vi "tcpserver.vi"   [LabVIEW 2016]
uses:
  executables/arguments.ctl
types:
  T1 = typedef "arguments.ctl" = cluster{"working directory":string, "flags":string[], "values":string[]}
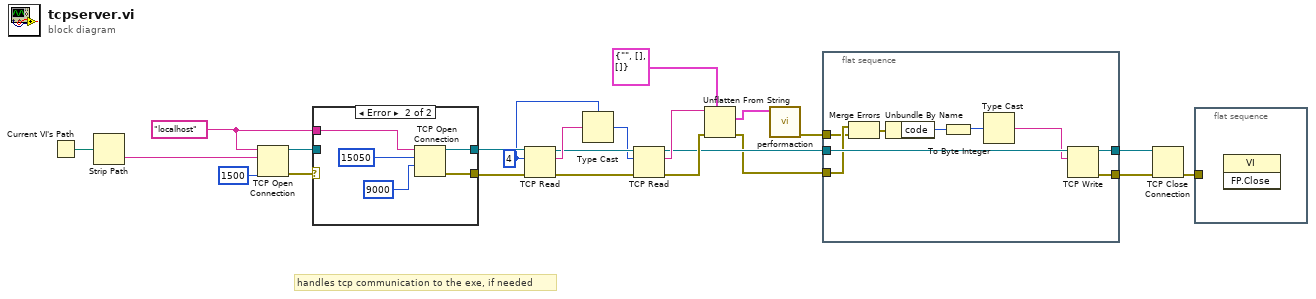
[diagram p0: block diagram]
diagram:
  w17 = 4 ("bytes to read")
  w20 = "localhost" ("address")
  # "handles tcp communication to the exe, if needed"
  n1 = Current VI's Path() -> (path=w3:path)
  n2 = Strip Path(path=w3) -> (name=w2:string)  [unwired: 1 out]
  n3 = TCP Open Connection(address=w20, remote port or service name=w2, timeout ms (60000)=1500) -> (connection ID=w21:refnum<k5>, error out=w22:errorcluster)  [unwired: 2 in]
  n4 = case shown="Error" w22 {
    selector: w22 -> [w24 _]
    tunnel: [w25 w30] -> w18
    tunnel: w21 -> [w25 _]
    tunnel: [w24 w29] -> w19
    tunnel: w20 -> [_ w28]
    frame No Error {
    }
    frame Error {
      n5 = TCP Open Connection(address=w28, remote port or service name=u16 15050 ("port"), timeout ms (60000)=9000) -> (connection ID=w30:refnum<k5>, error out=w29:errorcluster)  [unwired: 2 in]
    }
  }
  n6 = TCP Read(connection ID=w18, bytes to read=w17, error in (no error)=w19) -> (connection ID out=w15:refnum<k5>, data out=w16:string, error out=w14:errorcluster)  [unwired: 2 in]
  n7 = Type Cast(type=w17, x=w16) -> (*(type *) &x=w13:i32)
  n8 = TCP Read(connection ID=w15, bytes to read=w13, error in (no error)=w14) -> (connection ID out=w9:refnum<k5>, data out=w11:string, error out=w12:errorcluster)  [unwired: 2 in]
  n9 = Unflatten From String(type=T1 {"working directory"="", "flags"=[], "values"=[]} ("command line arguments"), binary string=w11, error in (no error)=w12) -> (value=w10:T1, error out=w5:errorcluster)  [unwired: 2 in, 1 out]
  n10 = call "performaction.vi"("command line arguments"=w10) -> ("error out"=w4:errorcluster)  [unwired: 10 in]
  n11 = flat-sequence {
    tunnel: w9 -> [w39]
    tunnel: [w38] -> w8
    tunnel: [w37] -> w7
    tunnel: w5 -> [w36]
    tunnel: w4 -> [w35]
    frame #0 {
      n12 = Merge Errors(w36, w35) -> (w34:errorcluster)
      n13 = Unbundle By Name(w34) -> ("code"=w33:i32)
      n14 = To Byte Integer(number=w33) -> (8bit integer=w32:i8)
      n15 = Type Cast(x=w32) -> (*(type *) &x=w31:string)  [unwired: 1 in]
      n16 = TCP Write(connection ID=w39, data in=w31) -> (connection ID out=w37:refnum<k5>, error out=w38:errorcluster)  [unwired: 2 in, 1 out]
    }
  }
  n17 = TCP Close Connection(connection ID=w7, error in (no error)=w8) -> (error out=w6:errorcluster)  [unwired: 1 in, 1 out]
  n18 = flat-sequence {
    tunnel: w6 -> [_]
    frame #0 {
      n19 = invoke class="VI" method="FP.Close"() -> ()  [unwired: 3 in, 3 out]
    }
  }
